vi "Read packed data from DRAM.vi"(11 "Output ready":bool) -> (2 "Output Valid§":bool, 3 "Data":T1)   [LabVIEW 2015]
uses:
  <vilib>/rvi/DataTransferAndStorage/Container/Common/niFpgaContainerGetUniqueNameForEmu.vi
  <vilib>/rvi/DataTransferAndStorage/Container/XNode/niFpgaContainer.xnode
  <vilib>/rvi/Memory/Memory_Emulation/niFpgaMemoryEmulationDramRetrieveData.vi
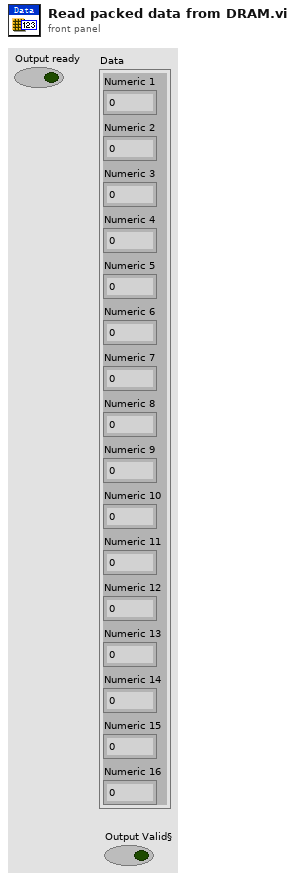
[diagram p1: front panel]
types:
  T1 = cluster{"Numeric 1":u32, "Numeric 2":u32, "Numeric 3":u32, "Numeric 4":u32, "Numeric 5":u32, "Numeric 6":u32, "Numeric 7":u32, "Numeric 8":u32, "Numeric 9":u32, "Numeric 10":u32, "Numeric 11":u32, "Numeric 12":u32, "Numeric 13":u32, "Numeric 14":u32, "Numeric 15":u32, "Numeric 16":u32}
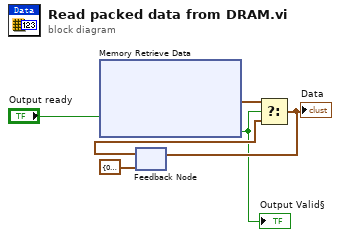
[diagram p0: block diagram]
diagram:
  n1 = xnode ("Memory Retrieve Data")("Ready for Output"="Output ready") -> ("Data"=w1:T1, "Output Valid"=w2:bool)  [unwired: 1 in, 1 out]
  "Output Valid§" <- w2
  n2 = feedback #1(T1 {"Numeric 1"=0, "Numeric 2"=0, "Numeric 3"=0, "Numeric 4"=0, "Numeric 5"=0, "Numeric 6"=0, "Numeric 7"=0, "Numeric 8"=0, "Numeric 9"=0, "Numeric 10"=0, "Numeric 11"=0, "Numeric 12"=0, "Numeric 13"=0, "Numeric 14"=0, "Numeric 15"=0, "Numeric 16"=0} ("Data")) -> (w3:T1)
  n3 = Select(t=w1, s=w2, f=w3) -> (s? t:f=w5:T1)
  "Data" <- w5
  n4 = feedback-in #1(w5) -> ()
